vi "(SubVI) Curve smooth.vi"(10 "Y":dbl[](array[numeric]), 11 "X":dbl[](array[numeric])) -> (2 "x + iy":cdb[](array[numeric]), 3 "Array":cluster{cdb[]}[](array[cluster]))   [LabVIEW 2016]
uses:
  <vilib>/Analysis/1siggen.llb/Ramp Pattern by Samples.vi
  <vilib>/gmath/NI_Gmath.lvlib
  <vilib>/Analysis/NI_AALBase.lvlib
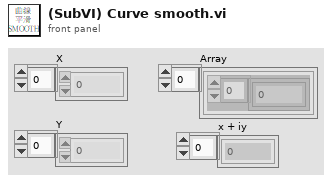
[diagram p1: front panel]
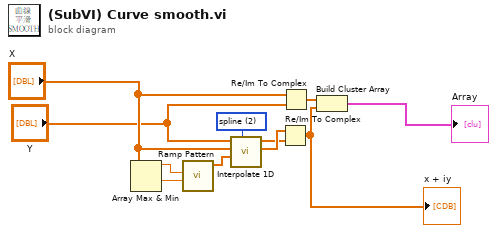
[diagram p0: block diagram]
diagram:
  w11 = 2 items=["nearest", "linear", "spline", "cubic Hermite", "Lagrange"] ("method")
  n1 = Array Max & Min(array="X") -> (max value=w5:dbl, min value=w4:dbl)  [unwired: 2 out]
  n2 = call-poly <vilib>:"Ramp Pattern.vi"("start"=w4, "end"=w5) -> ("Ramp Pattern"=w6:dbl[])  [unwired: 8 in, 1 out]
  n3 = call <vilib>:"Interpolate 1D.vi"("method"=w11, "xi"=w6, "X"="X", "Y"="Y") -> ("xi used"=w8:dbl[], "yi"=w7:dbl[])  [unwired: 5 in, 1 out]
  n4 = Re/Im To Complex(1:w7, 2:w8) -> (0:w10:cdb[])
  "x + iy" <- w10
  n5 = Re/Im To Complex(1:"Y", 2:"X") -> (0:w1:cdb[])
  n6 = Build Cluster Array(w1, w10) -> (→"Array":cluster{cdb[]}[])
